vi "Discover Unique Names of Dependencies.vi"(0 "NSIS_Installer In":refnum<class "Compound_Installer.lvclass">) -> (4 "NSIS_Installer Out":refnum<class "Compound_Installer.lvclass">)   [LabVIEW 2017, in "CL_G3_VIComponentBuilder.lvlib" / "Compound_Installer.lvclass"]
doc: "Interrogates this exports dependencies for thier unique names (as opposed to the product name of the dependency). The unique names are used when assembling the working set of exports in order to prevent name collisions and allow the build analyzer to determine the build order."
uses:
  Compound_Installer.lvclass
  Exports/Export.lvclass
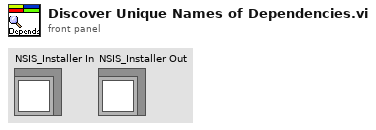
[diagram p1: front panel]
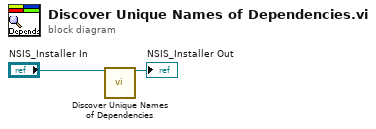
[diagram p0: block diagram]
diagram:
  n1 = call-parent "Discover Unique Names of Dependencies.vi"("Export In"="NSIS_Installer In") -> ("Export Out"=→"NSIS_Installer Out":refnum<class "Compound_Installer.lvclass">)  [unwired: 14 in]
